vi "Teleop.vi"(10 "Match Info":T1={"Autonomous Elapsed Seconds"=0.0, "TeleOp Elapsed Seconds"=0.0, "Disabled Elapsed Seconds"=0.0, "Visited Autonomous"=FALSE, "Visited TeleOp"=FALSE, "Visited Disabled"=FALSE, "Autonomous Settings"={"Autonomous Style"=enum."Independent", "VI Refnum"=refnum}}, 11 "Call Context":T2) -> ()   [LabVIEW 2013]
doc: "This VI is called for each TeleOp packet received from the DS where the robot is not disabled. It is often used to read from the joysticks and update I/O or to update setpoints for timed control loops. It should complete and return within 20 milliseconds or it may miss DS packets."
uses:
  <vilib>/Rock Robotics/WPI/DriverStation/WPI_DriverStationDerivedRobotMode.ctl
  <vilib>/Rock Robotics/WPI/DriverStation/WPI_DriverStationMatch Info.ctl
  <vilib>/Rock Robotics/WPI/Solenoid/WPI_SolenoidValue.ctl
  Robot Global Data.vi
  <vilib>/Rock Robotics/WPI/Solenoid/WPI_SolenoidSetEnum.vi
  <vilib>/Rock Robotics/WPI/RobotDrive/WPI_RobotDriveMecanumDrive_Cartesian.vi
  <vilib>/Rock Robotics/WPI/Joystick/WPI_JoystickGetSetRefNum.vi
  <vilib>/Rock Robotics/WPI/Compressor/WPI_CompressorGetSetRefNum.vi
  <vilib>/Rock Robotics/WPI/RobotDrive/WPI_RobotDriveGetSetRefNum.vi
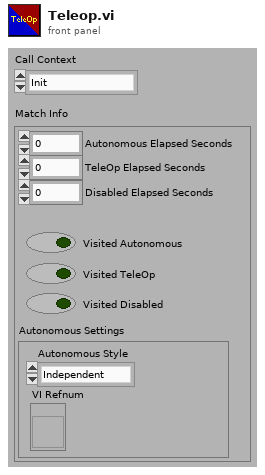
[diagram p1: front panel]
types:
  T1 = typedef "WPI_DriverStationMatch Info.ctl" = cluster{"Autonomous Elapsed Seconds":dbl, "TeleOp Elapsed Seconds":dbl, "Disabled Elapsed Seconds":dbl, "Visited Autonomous":bool, "Visited TeleOp":bool, "Visited Disabled":bool, "Autonomous Settings":cluster{"Autonomous Style":enum16{"Iterative", "Independent"}, "VI Refnum":refnum<vi>}}
  T2 = typedef "WPI_DriverStationDerivedRobotMode.ctl" = enum16{"Init", "Execute", "Stop"}
  T3 = typedef "WPI_SolenoidValue.ctl" = enum16{"Off", "On", "Forward", "Reverse"}
  T4 = typedef "WPI_RobotDriveDevRef.ctl" = cluster{"DevStatus":errorcluster, "Motors[]":T5[], "Square Inputs":bool, "Max Output":dbl, "Isochronous":bool}
  T5 = typedef "WPI_MotorControlDeviceRef.ctl" = cluster{"DeviceStatus":errorcluster, "Type":enum16{"PWM", "CAN"}, "PWM":cluster{"Digital Module":T6, "PWM Channel":T7, "DeadBand":T8}, "CAN":cluster{"Device Number":u8, "Control Mode":T9, "Semaphore":T10, "Max Vout":dbl}, "Invert":bool, "TransformRef":T11, "InvTransformRef":T11}
  T6 = typedef "FPGA_TypedefDigitalModule.ctl" = enum16{"Digital Module 1", "Digital Module 2"}
  T7 = typedef "FPGA_DIOPWMChannel.ctl" = enum8{"PWM 1", "PWM 2", "PWM 3", "PWM 4", "PWM 5", "PWM 6", "PWM 7", "PWM 8", "PWM 9", "PWM 10", "Invalid"}
  T8 = typedef "WPI_PWMDeadband.ctl" = cluster{"Name":string, "maxPositivePwm":i32, "minPositivePwm":i32, "centerPwm":i32, "maxNegativePwm":i32, "minNegativePwm":i32, "angularRange":u16}
  T9 = typedef "WPI_CANJaguar_ControlMode.ctl" = enum8{"Percent VBus", "Current", "Speed", "Position", "Voltage"}
  T10 = typedef "Semaphore RefNum" = refnum<k1>
  T11 = typedef "WPI_PWMTransform_ConPane.ctl" = refnum<vi>
  T12 = typedef "WPI_JoystickDevRef.ctl" = cluster{"Device":T13}
  T13 = typedef "WPI_JoystickDeviceEnum.ctl" = enum16{"USB 1", "USB 2", "USB 3", "USB 4", "Kinect 1", "Kinect 2"}
  T14 = typedef "WPI_CompressorDevRef.ctl" = cluster{"DevStatus":errorcluster, "DigitalInputDevRef":T15, "RelayDevRef":T17}
  T15 = typedef "WPI_DigitalInputDevRef.ctl" = cluster{"DevStatus":errorcluster, "DIO Channel":T16, "Digital Module":T6}
  T16 = typedef "FPGA_DIOChannel.ctl" = enum8{"DIO 1", "DIO 2", "DIO 3", "DIO 4", "DIO 5", "DIO 6", "DIO 7", "DIO 8", "DIO 9", "DIO 10", "DIO 11", "DIO 12", "DIO 13", "DIO 14", "Invalid"}
  T17 = typedef "WPI_RelayDevRef.ctl" = cluster{"DevStatus":errorcluster, "Relay Channel":T18, "Digital Module":T6, "Relay Direction":T19}
  T18 = typedef "FPGA_DIORelayChannel.ctl" = enum8{"Relay 1", "Relay 2", "Relay 3", "Relay 4", "Relay 5", "Relay 6", "Relay 7", "Relay 8", "Invalid"}
  T19 = typedef "WPI_RelayDirection.ctl" = enum16{"Both directions", "Forward only", "Reverse only"}
  T20 = typedef "WPI_JoystickButtonState.ctl" = cluster{"Button 1":bool, "Button 2":bool, "Button 3":bool, "Button 4":bool, "Button 5":bool, "Button 6":bool, "Button 7":bool, "Button 8":bool, "Button 9":bool, "Button 10":bool, "Button 11":bool, "Button 12":bool}
  T21 = cluster{"axis 1 (x)":dbl, "axis 2 (y)":dbl, "axis 3 (throttle)":dbl, "axis 4":dbl, "axis 5":dbl, "axis 6":dbl}
  T22 = typedef "WPI_SolenoidDevRef.ctl" = cluster{"DevStatus":errorcluster, "Solenoid Module":T23, "Forward Solenoid Channel":T24, "Reverse Solenoid Channel":T24}
  T23 = typedef "FPGA_TypedefSolenoidModule.ctl" = enum16{"Solenoid Module 1", "Solenoid Module 2"}
  T24 = typedef "WPI_SolenoidChannel.ctl" = enum8{"Solenoid 1", "Solenoid 2", "Solenoid 3", "Solenoid 4", "Solenoid 5", "Solenoid 6", "Solenoid 7", "Solenoid 8", "Invalid"}
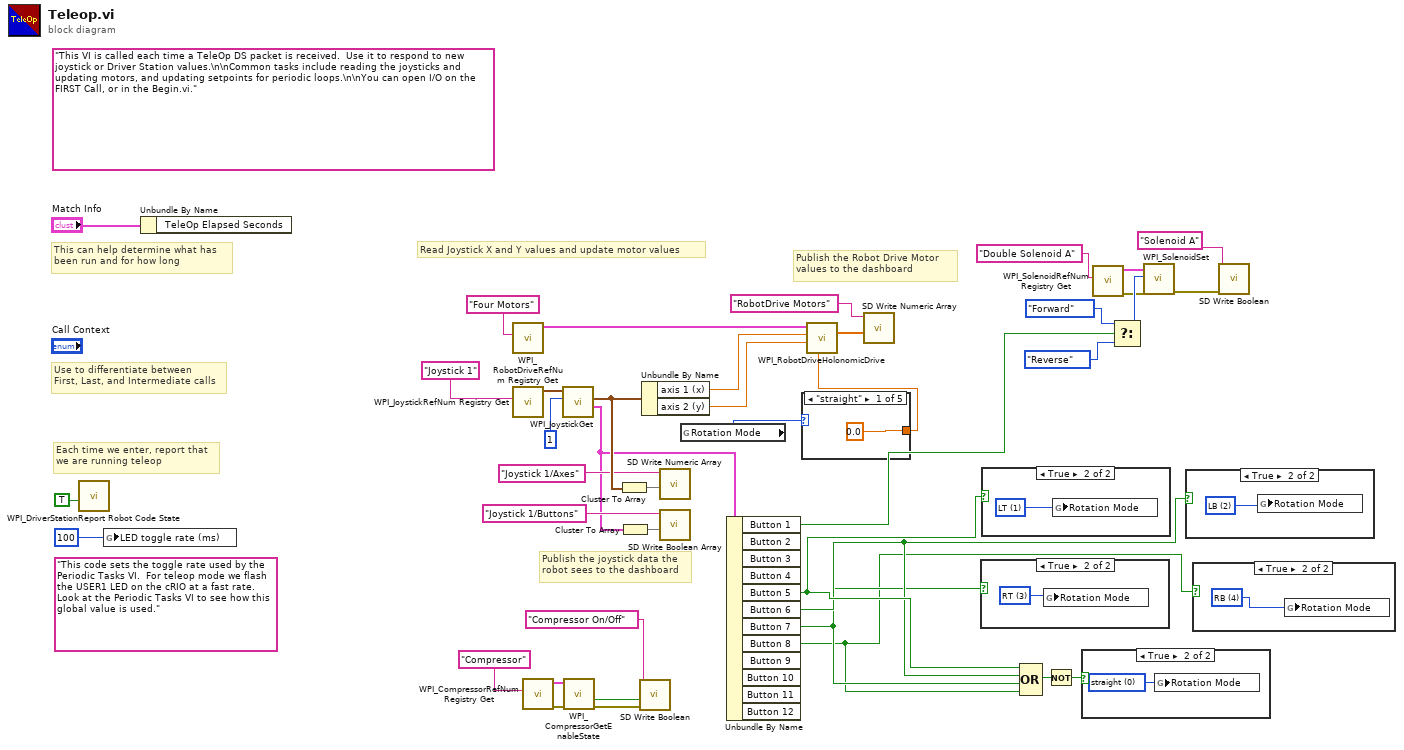
[diagram p0: block diagram]
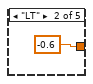
[diagram p2: hidden frame]
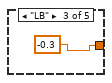
[diagram p3: hidden frame]
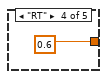
[diagram p4: hidden frame]
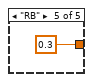
[diagram p5: hidden frame]
diagram:
  (unwired) "This code sets the toggle rate used by the Periodic Tasks VI.  For teleop mode we flash the USER1 LED on the cRIO at a fast rate.  Look at the Periodic Tasks VI to see how this global value is used."
  (unwired) "This VI is called each time a TeleOp DS packet is received.  Use it to respond to new joystick or Driver Station values.\n\nCommon tasks include reading the joysticks and updating motors, and updating setpoints for periodic loops.\n\nYou can open I/O on the FIRST Call, or in the Begin.vi."
  # "Publish the Robot Drive Motor\nvalues to the dashboard"
  # "Publish the joystick data the\nrobot sees to the dashboard"
  # "Each time we enter, report that\nwe are running teleop"
  # "Use to differentiate between\nFirst, Last, and Intermediate calls"
  # "This can help determine what has\nbeen run and for how long"
  # "Read Joystick X and Y values and update motor values"
  n1 = call <vilib>:"WPI_DriverStationReport Robot Code State.vi"("TeleOp"=TRUE ("Autonomous")) -> ()  [unwired: 10 in, 1 out]
  n2 = global write "Robot Global Data.vi" "LED toggle rate (ms)"(u32 100 ("LED ms toggle rate")) -> ()
  n3 = Unbundle By Name("Match Info") -> ()  [unwired: 1 out]
  n4 = call <vilib>:"WPI_RobotDriveRefNum Registry Get.vi"("refnum name"="Four Motors") -> ("RobotDriveDevRef"=w39:T4)  [unwired: 1 in, 9 out]
  n5 = call <vilib>:"WPI_JoystickRefNum Registry Get.vi"("refnum name"="Joystick 1") -> ("JoystickDevRef"=w35:T12)  [unwired: 1 in, 9 out]
  n6 = call <vilib>:"WPI_CompressorRefNum Registry Get.vi"("refnum name"="Compressor") -> ("error out"=w25:errorcluster, "CompressorDevRef"=w24:T14)  [unwired: 9 in]
  n7 = call <vilib>:"WPI_JoystickGet.vi"("Scaler"=1, "JoystickDevRef"=w35) -> ("Buttons"=w11:T20, "Axes"=w30:T21)  [unwired: 4 out]
  n8 = call <vilib>:"WPI_CompressorGetEnableState.vi"("error in (no error)"=w25, "CompressorDevRef"=w24) -> ("error out"=w18:errorcluster, "Compressor Running"=w17:bool)  [unwired: 6 in, 2 out]
  n9 = Cluster To Array(cluster=w30) -> (array=w29:dbl[])
  n10 = Cluster To Array(cluster=w11) -> (array=w32:bool[])
  n11 = call <vilib>:"SD Write Boolean.vi"("error in"=w18, "Boolean"=w17, "Name"="Compressor On/Off") -> ()  [unwired: 7 in, 2 out]
  n12 = Unbundle By Name(w30) -> ("axis 1 (x)"=w38:dbl, "axis 2 (y)"=w37:dbl)
  n13 = call <vilib>:"SD Write Numeric Array.vi"("Numeric Array"=w29, "Name"="Joystick 1/Axes") -> ()  [unwired: 8 in, 2 out]
  n14 = call <vilib>:"SD Write Boolean Array.vi"("Boolean Array"=w32, "Name"="Joystick 1/Buttons") -> ()  [unwired: 8 in, 2 out]
  n15 = global read "Robot Global Data.vi" "Rotation Mode"() -> (w2:enum16{"straight", "LT", "LB", "RT", "RB"})
  n16 = Unbundle By Name(w11) -> ("Button 1"=w12:bool, "Button 5"=w7:bool, "Button 6"=w6:bool, "Button 7"=w5:bool, "Button 8"=w4:bool)  [unwired: 7 out]
  n17 = case shown="\"straight\"" w2 {
    tunnel: [0.0 -0.6 -0.3 0.6 0.3] -> w1
    frame "straight" {
    }
    frame "LT" {
    }
    frame "LB" {
    }
    frame "RT" {
    }
    frame "RB" {
    }
  }
  n18 = call-poly <vilib>:"WPI_RobotDriveHolonomicDrive.vi"("Rotation"=w1, "Y"=w37, "X"=w38, "RobotDriveDevRef"=w39) -> ("Motor Values"=w26:dbl[])  [unwired: 5 in, 2 out]
  n19 = call <vilib>:"SD Write Numeric Array.vi"("Numeric Array"=w26, "Name"="RobotDrive Motors") -> ()  [unwired: 8 in, 2 out]
  n20 = case shown="True" w5 {
    frame False {
    }
    frame True {
      w47 = u16 3 items=["straight", "LT", "LB", "RT", "RB"]
      n21 = global write "Robot Global Data.vi" "Rotation Mode"(w47) -> ()
    }
  }
  n22 = case shown="True" w7 {
    frame False {
    }
    frame True {
      w48 = u16 1 items=["straight", "LT", "LB", "RT", "RB"]
      n23 = global write "Robot Global Data.vi" "Rotation Mode"(w48) -> ()
    }
  }
  n24 = Compound Arithmetic op=OR(w7, w6, w5, w4) -> (w8:bool)
  n25 = Not(x=w8) -> (.not. x?=w9:bool)
  n26 = case shown="True" w9 {
    frame False {
    }
    frame True {
      w49 = u16 0 items=["straight", "LT", "LB", "RT", "RB"]
      n27 = global write "Robot Global Data.vi" "Rotation Mode"(w49) -> ()
    }
  }
  n28 = call <vilib>:"WPI_SolenoidRefNum Registry Get.vi"("refnum name"="Double Solenoid A") -> ("error out"=w15:errorcluster, "SolenoidDevRef"=w21:T22)  [unwired: 9 in]
  n29 = Select(t=WPI_SolenoidValue."Forward" ("Value"), s=w12, f=WPI_SolenoidValue."Reverse" ("Value")) -> (s? t:f=w19:T3)
  n30 = call-poly <vilib>:"WPI_SolenoidSet.vi"("error in (no error)"=w15, "Value"=w19, "SolenoidDevRef"=w21) -> ("error out"=w14:errorcluster)  [unwired: 7 in, 1 out]
  n31 = case shown="True" w6 {
    frame False {
    }
    frame True {
      w50 = u16 2 items=["straight", "LT", "LB", "RT", "RB"]
      n32 = global write "Robot Global Data.vi" "Rotation Mode"(w50) -> ()
    }
  }
  n33 = case shown="True" w4 {
    frame False {
    }
    frame True {
      w51 = u16 4 items=["straight", "LT", "LB", "RT", "RB"]
      n34 = global write "Robot Global Data.vi" "Rotation Mode"(w51) -> ()
    }
  }
  n35 = call <vilib>:"SD Write Boolean.vi"("error in"=w14, "Name"="Solenoid A") -> ()  [unwired: 8 in, 2 out]
